vi "Init.vi"(8 "error in":errorcluster, 11 "ColumnHeader View in":refnum<class "ColumnHeader View.lvclass">) -> (0 "error out":errorcluster, 3 "ColumnHeader View out":refnum<class "ColumnHeader View.lvclass">)   [LabVIEW 2024, in "SourceGrid.lvlib" / "ColumnHeader View.lvclass"]
uses:
  ColumnHeader View.lvclass
  Cell View/Cell View.lvclass/Cell View.ctl
  D:/git/Sourcegrid-LabVIEW/dll/SourceGrid.dll
  dll/SourceGrid.dll
  ColumnHeader View.lvclass/ColumnHeader View.ctl
  Cell View/Cell View.lvclass
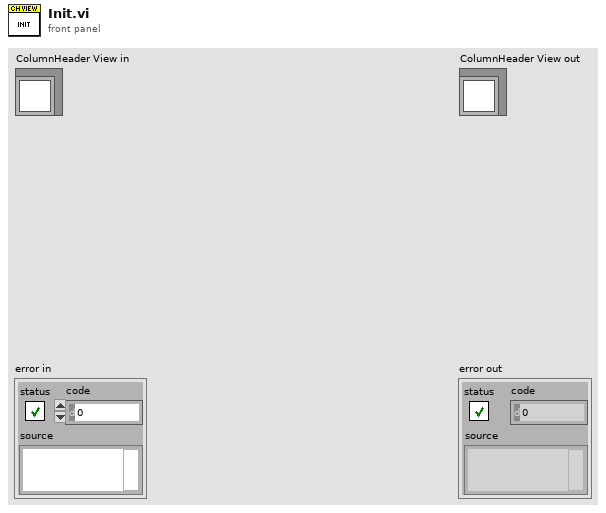
[diagram p1: front panel]
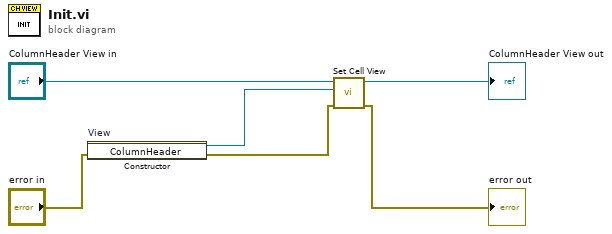
[diagram p0: block diagram]
diagram:
  n1 = constructor on="View" class="ColumnHeader"(error in="error in") -> (reference out=w4:refnum<k24>, error out=w3:errorcluster)  [unwired: 2 in, 1 out]
  n2 = call "Set Cell View.vi"("error in (no error)"=w3, "Cell View"=w4, "Cell View in"="ColumnHeader View in") -> ("error out"=→"error out":errorcluster, "Cell View out"=→"ColumnHeader View out":refnum<class "ColumnHeader View.lvclass">)  [unwired: 7 in]
